vi "Autonomous Independent.vi"() -> ()   [LabVIEW 2017]
doc: "This VI is called when autonomous begins, and will automatically be terminated when autonomous ends. You can carry out timed or sensor driven robot movement independently without needing to return to the caller."
uses:
  <vilib>/Rock Robotics/WPI/Solenoid/WPI_SolenoidValue.ctl
  <vilib>/Rock Robotics/Network Tables/NT Read String.vi
  <vilib>/Rock Robotics/Network Tables/NT Read Numeric Array.vi
  <vilib>/Rock Robotics/Network Tables/NT Read String Array.vi
  <vilib>/Rock Robotics/WPI/Solenoid/WPI_SolenoidSetEnum.vi
  Robot Global Data.vi
panel:
  out "Setpoint2":dbl
  out "Setpoint":dbl
  in  "Z Drive PID Gains":T1
  # "Be sure to right-click and choose Data Operations>>Make Current Value default if you want to save the array values with the VI"
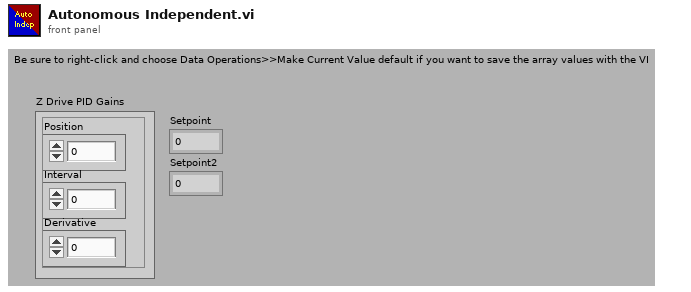
[diagram p1: front panel]
types:
  T1 = cluster{"Position":dbl, "Interval":dbl, "Derivative":dbl}
  T2 = typedef "WPI_SolenoidValue.ctl" = enum16{"Off", "On", "Forward", "Reverse"}
  T3 = enum16{"Front Left", "Front Right", "Back Left", "Back Right"}
  T4 = typedef "WPI_SolenoidDevRef.ctl" = cluster{"DevStatus":errorcluster, "Pneumatics Control Module":u8, "Forward Solenoid Channel":T5, "Reverse Solenoid Channel":T5}
  T5 = typedef "WPI_SolenoidChannel.ctl" = enum8{"Solenoid 0", "Solenoid 1", "Solenoid 2", "Solenoid 3", "Solenoid 4", "Solenoid 5", "Solenoid 6", "Solenoid 7", "Invalid"}
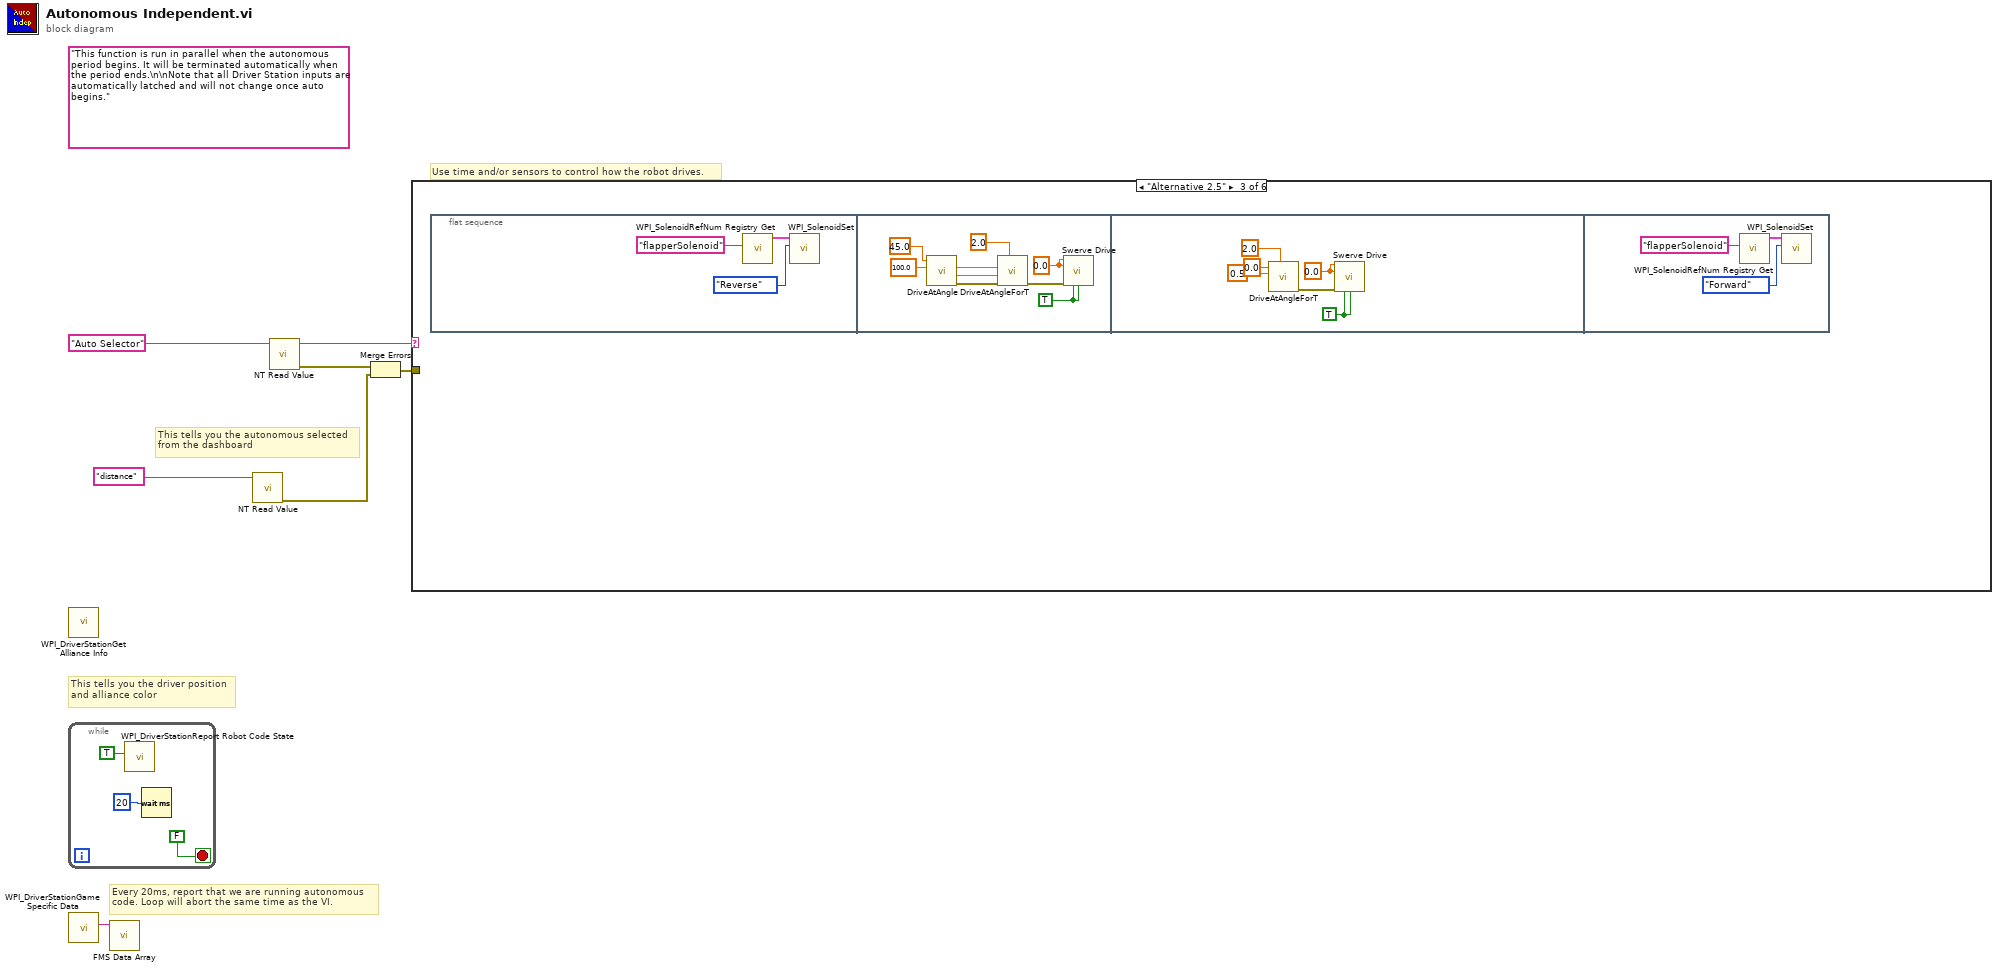
[diagram p0: block diagram]
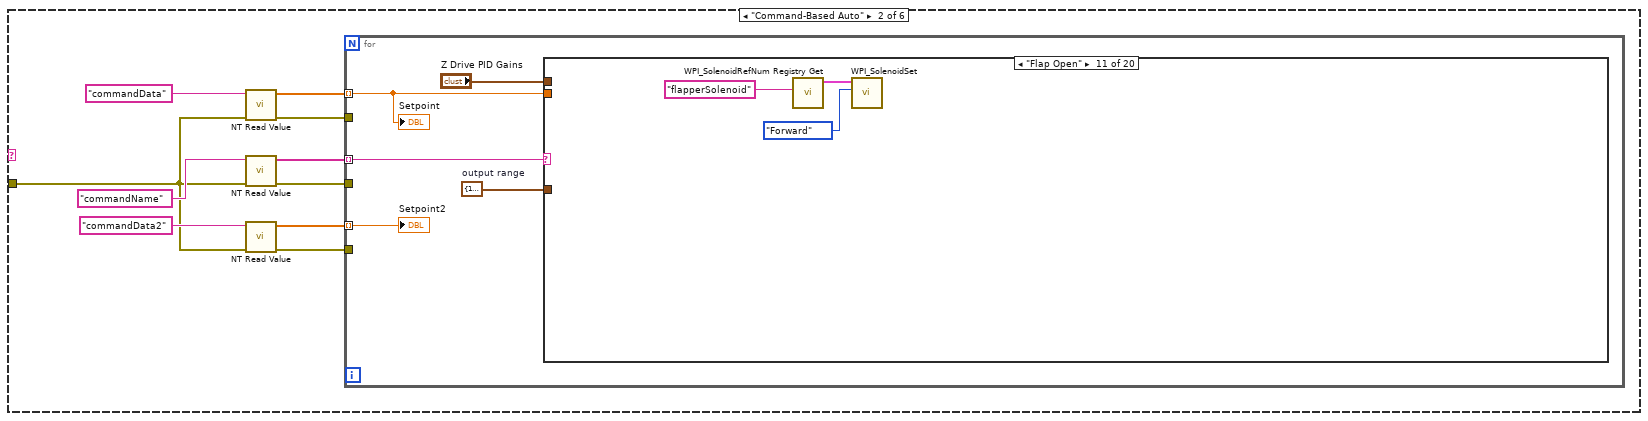
[diagram p3: hidden frame]
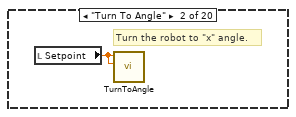
[diagram p5: hidden frame]
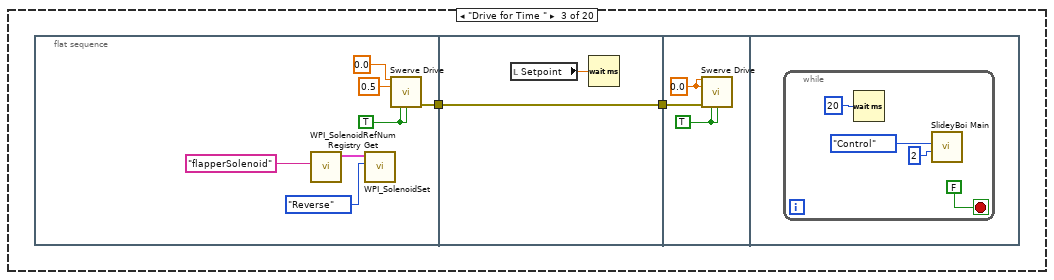
[diagram p6: hidden frame]
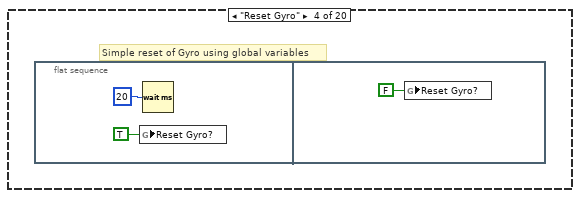
[diagram p7: hidden frame]
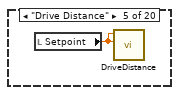
[diagram p8: hidden frame]
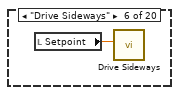
[diagram p9: hidden frame]
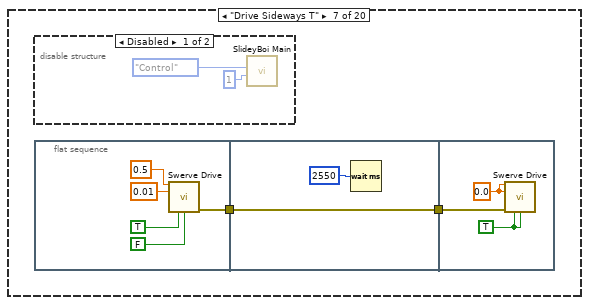
[diagram p10: hidden frame]
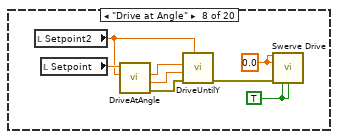
[diagram p12: hidden frame]
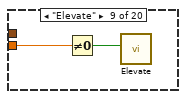
[diagram p13: hidden frame]
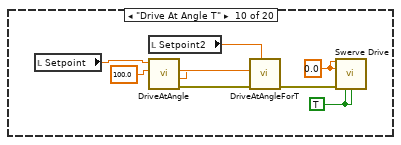
[diagram p14: hidden frame]
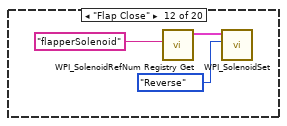
[diagram p15: hidden frame]
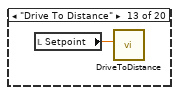
[diagram p16: hidden frame]
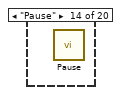
[diagram p17: hidden frame]
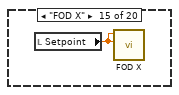
[diagram p18: hidden frame]
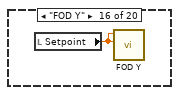
[diagram p19: hidden frame]
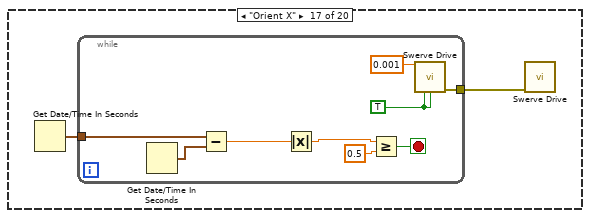
[diagram p20: hidden frame]
diagram:
  (unwired) "This function is run in parallel when the autonomous period begins. It will be terminated automatically when the period ends.\n\nNote that all Driver Station inputs are automatically latched and will not change once auto begins."
  # "This tells you the autonomous selected\nfrom the dashboard"
  # "Every 20ms, report that we are running autonomous\ncode. Loop will abort the same time as the VI."
  # "Use time and/or sensors to control how the robot drives."
  # "This tells you the driver position\nand alliance color"
  n1 = call <vilib>:"WPI_DriverStationGet Alliance Info.vi"() -> ()  [unwired: 12 out]
  n2 = while {
    stop <- FALSE stop-if-true
    n3 = call <vilib>:"WPI_DriverStationReport Robot Code State.vi"("Autonomous"=TRUE) -> ()  [unwired: 10 in, 1 out]
    n4 = Wait (ms)(milliseconds to wait=u32 20) -> ()  [unwired: 1 out]
  }
  n5 = call <vilib>:"WPI_DriverStationGame Specific Data.vi"() -> ("Game Specific Data"=w5:string)  [unwired: 11 in]
  n6 = call "FMS Data Array.vi"("Game Data"=w5) -> ()  [unwired: 8 in, 3 out]
  n7 = call-poly <vilib>:"NT Read Value.vi"("Name"="distance") -> ("error out"=w3:errorcluster)  [unwired: 9 in, 1 out]
  n8 = call-poly <vilib>:"NT Read Value.vi"("Name"="Auto Selector") -> ("error out"=w4:errorcluster, "String"=w6:string)  [unwired: 9 in]
  n9 = Merge Errors(w4, w3) -> (w1:errorcluster)
  n10 = case shown="\"Alternative 2.5\"" w6 {
    tunnel: w1 -> [_ w11 _ _ _ _]
    frame Default {
      # "You can put your main auto here, or you can right-click on the case and make any\nother frame be the default case."
      # "This is the frame that will execute if no selection is made, or if it is not recognized"
    }
    frame "Command-Based Auto" {
      n11 = call-poly <vilib>:"NT Read Value.vi"("error in"=w11, "Name"="commandData") -> ("error out"=w18:errorcluster, "Numeric Array"=w15:dbl[])  [unwired: 8 in]
      n12 = call-poly <vilib>:"NT Read Value.vi"("error in"=w11, "Name"="commandName") -> ("error out"=w17:errorcluster, "String Array"=w16:string[])  [unwired: 8 in]
      n13 = call-poly <vilib>:"NT Read Value.vi"("error in"=w11, "Name"="commandData2") -> ("error out"=w14:errorcluster, "Numeric Array"=w13:dbl[])  [unwired: 8 in]
      n14 = for {
        tunnel: w18 -> [_]
        tunnel: w17 -> [_]
        tunnel: w16 -> [w25] mode=indexing
        tunnel: w15 -> [w21] mode=indexing
        tunnel: w14 -> [_]
        tunnel: w13 -> [w24] mode=indexing
        w22 = cluster{dbl, dbl} {1.0, -1.0}  # output range
        n15 = case shown="\"Flap Open\"" w25 {
          tunnel: "Z Drive PID Gains" -> [_ _ _ _ _ _ _ _ _ _ _ _ _ _ _ _ _ _ _ _]
          tunnel: w22 -> [_ _ _ _ _ _ _ _ _ _ _ _ _ _ _ _ _ _ _ _]
          tunnel: w21 -> [_ _ _ _ _ _ _ _ w73 _ _ _ _ _ _ _ _ _ _ _]
          frame Default {
          }
          frame "Turn To Angle" {
            # "Turn the robot to \"x\" angle."
            n16 = local read "Setpoint"() -> (w26:dbl)
            n17 = call "TurnToAngle.vi"(10:"Target Angle"=w26, 11:"Target Angle"=w26) -> ()  [unwired: 9 in, 1 out]
          }
          frame "Drive for Time " {
            n18 = flat-sequence {
              tunnel: [w32] -> w28
              tunnel: [w37] -> w27
              tunnel: w28 -> [w37]
              tunnel: w27 -> [w39]
              frame #0 {
                w33 = TRUE ("Autonomous?")
                n19 = call <vilib>:"WPI_SolenoidRefNum Registry Get.vi"("refnum name"="flapperSolenoid") -> ("SolenoidDevRef"=w31:T4)  [unwired: 9 in, 1 out]
                n20 = call-poly <vilib>:"WPI_SolenoidSet.vi"("Value"=WPI_SolenoidValue."Reverse", "SolenoidDevRef"=w31) -> ()  [unwired: 8 in, 2 out]
                n21 = call "Swerve Drive.vi"("X"=0.0, "Y"=0.5, "Robot Centric?"=w33, "Autonomous?"=w33) -> ("Error Out"=w32:errorcluster)  [unwired: 7 in, 4 out]
              }
              frame #1 {
                n22 = local read "Setpoint"() -> (w36:dbl)
                n23 = Wait (ms)(milliseconds to wait=w36) -> ()  [unwired: 1 out]
              }
              frame #2 {
                w38 = TRUE ("Robot Centric?")
                w40 = 0.0 ("X")
                n24 = call "Swerve Drive.vi"("X"=w40, "Y"=w40, "Error In"=w39, "Robot Centric?"=w38, "Autonomous?"=w38) -> ()  [unwired: 6 in, 5 out]
              }
              frame #3 {
                n25 = while {
                  stop <- FALSE stop-if-true
                  n26 = Wait (ms)(milliseconds to wait=u32 20) -> ()  [unwired: 1 out]
                  n27 = call "SlideyBoi Main.vi"("Control Option"=u32 2, "Control Mode"=enum16{"Open", "Control"}."Control") -> ()  [unwired: 10 in]
                }
              }
            }
          }
          frame "Reset Gyro" {
            # "Simple reset of Gyro using global variables"
            n28 = flat-sequence {
              frame #0 {
                n29 = global write "Robot Global Data.vi" "Reset Gyro?"(TRUE ("Enable Vision")) -> ()
                n30 = Wait (ms)(milliseconds to wait=u32 20) -> ()  [unwired: 1 out]
              }
              frame #1 {
                n31 = global write "Robot Global Data.vi" "Reset Gyro?"(FALSE ("Reset Gyro?")) -> ()
              }
            }
          }
          frame "Drive Distance" {
            n32 = local read "Setpoint"() -> (w48:dbl)
            n33 = call "DriveDistance.vi"(10:"Setpoint"=w48, 11:"Setpoint"=w48) -> ()  [unwired: 10 in]
          }
          frame "Drive Sideways" {
            n34 = local read "Setpoint"() -> (w49:dbl)
            n35 = call "Drive Sideways.vi"("Setpoint"=w49) -> ()  [unwired: 10 in]
          }
          frame "Drive Sideways T" {
            n36 = disable-structure shown="Disabled" {
              frame Disabled {
                n37 = call "SlideyBoi Main.vi"("Control Option"=u32 1, "Control Mode"=enum16{"Open", "Control"}."Control") -> ()  [unwired: 10 in]
              }
              frame Enabled {
              }
            }
            n38 = flat-sequence {
              tunnel: [w55] -> w51
              tunnel: w51 -> [w59]
              tunnel: [w59] -> w50
              tunnel: w50 -> [w61]
              frame #0 {
                n39 = call "Swerve Drive.vi"("X"=0.5, "Y"=0.01, "Robot Centric?"=TRUE, "Autonomous?"=FALSE) -> ("Error Out"=w55:errorcluster)  [unwired: 7 in, 4 out]
              }
              frame #1 {
                n40 = Wait (ms)(milliseconds to wait=u32 2550) -> ()  [unwired: 1 out]
              }
              frame #2 {
                w62 = TRUE
                w63 = 0.0 ("X")
                n41 = call "Swerve Drive.vi"("X"=w63, "Y"=w63, "Error In"=w61, "Robot Centric?"=w62, "Autonomous?"=w62) -> ()  [unwired: 6 in, 5 out]
              }
            }
          }
          frame "Drive at Angle" {
            w65 = TRUE ("Robot Centric?")
            w70 = 0.0 ("X")
            n42 = local read "Setpoint2"() -> (w64:dbl)
            n43 = local read "Setpoint"() -> (w68:dbl)
            n44 = call "DriveAtAngle.vi"("Target Angle"=w68, "Distance"=w64) -> ("x"=w66:dbl, "y"=w67:dbl, "Error Out"=w71:errorcluster)  [unwired: 5 in, 1 out]
            n45 = call "DriveUntilY.vi"("Stop  Distance"=w64, "error in"=w71, "y"=w67, "x"=w66) -> ("error out"=w69:errorcluster)  [unwired: 7 in]
            n46 = call "Swerve Drive.vi"("X"=w70, "Y"=w70, "Error In"=w69, "Robot Centric?"=w65, "Autonomous?"=w65) -> ()  [unwired: 6 in, 5 out]
          }
          frame "Elevate" {
            n47 = Not Equal To 0?(x=w73) -> (x != 0?=w72:bool)
            n48 = call "Elevate.vi"("Reverse"=w72) -> ()  [unwired: 11 in]
          }
          frame "Drive At Angle T" {
            w78 = 0.0 ("X")
            w77 = TRUE ("Robot Centric?")
            n49 = local read "Setpoint"() -> (w82:dbl)
            n50 = local read "Setpoint2"() -> (w76:dbl)
            n51 = call "DriveAtAngle.vi"("Target Angle"=w82, "Distance"=100.0) -> ("x"=w81:dbl, "y"=w80:dbl, "Error Out"=w75:errorcluster)  [unwired: 5 in, 1 out]
            n52 = call "DriveAtAngleForT.vi"("time(sec)"=w76, "Error In"=w75, "y"=w80, "x"=w81) -> ("Error Out"=w79:errorcluster)  [unwired: 7 in]
            n53 = call "Swerve Drive.vi"("X"=w78, "Y"=w78, "Error In"=w79, "Robot Centric?"=w77, "Autonomous?"=w77) -> ()  [unwired: 6 in, 5 out]
          }
          frame "Flap Open" {
            n54 = call <vilib>:"WPI_SolenoidRefNum Registry Get.vi"("refnum name"="flapperSolenoid") -> ("SolenoidDevRef"=w84:T4)  [unwired: 9 in, 1 out]
            n55 = call-poly <vilib>:"WPI_SolenoidSet.vi"("Value"=WPI_SolenoidValue."Forward", "SolenoidDevRef"=w84) -> ()  [unwired: 8 in, 2 out]
          }
          frame "Flap Close" {
            n56 = call <vilib>:"WPI_SolenoidRefNum Registry Get.vi"("refnum name"="flapperSolenoid") -> ("SolenoidDevRef"=w88:T4)  [unwired: 9 in, 1 out]
            n57 = call-poly <vilib>:"WPI_SolenoidSet.vi"("Value"=WPI_SolenoidValue."Reverse", "SolenoidDevRef"=w88) -> ()  [unwired: 8 in, 2 out]
          }
          frame "Drive To Distance" {
            n58 = local read "Setpoint"() -> (w89:dbl)
            n59 = call "DriveToDistance.vi"("Setpoint"=w89) -> ()  [unwired: 10 in, 1 out]
          }
          frame "Pause" {
            n60 = call "Pause.vi"() -> ()  [unwired: 11 in, 1 out]
          }
          frame "FOD X" {
            n61 = local read "Setpoint"() -> (w90:dbl)
            n62 = call "FOD X.vi"(10:"Setpoint"=w90, 11:"Setpoint"=w90) -> ()  [unwired: 10 in]
          }
          frame "FOD Y" {
            n63 = local read "Setpoint"() -> (w91:dbl)
            n64 = call "FOD Y.vi"(10:"Setpoint"=w91, 11:"Setpoint"=w91) -> ()  [unwired: 10 in]
          }
          frame "Orient X" {
            n65 = Get Date/Time In Seconds() -> (seconds since 1Jan1904=w93:timestamp)
            n66 = while {
              tunnel: w93 -> [w101]
              tunnel: [w96] -> w92
              stop <- w97 stop-if-true
              w94 = TRUE ("Robot Centric?")
              n67 = Get Date/Time In Seconds() -> (seconds since 1Jan1904=w102:timestamp)
              n68 = Subtract(x=w101, y=w102) -> (x-y=w100:dbl)
              n69 = Absolute Value(x=w100) -> (abs(x)=w99:dbl)
              n70 = Greater Or Equal?(x=w99, y=0.5) -> (x >= y?=w97:bool)
              n71 = call "Swerve Drive.vi"("X"=0.001, "Robot Centric?"=w94, "Autonomous?"=w94) -> ("Error Out"=w96:errorcluster)  [unwired: 8 in, 4 out]
            }
            n72 = call "Swerve Drive.vi"("Error In"=w92) -> ()  [unwired: 10 in, 5 out]
          }
          frame "Orient Y" {
            n73 = Get Date/Time In Seconds() -> (seconds since 1Jan1904=w104:timestamp)
            n74 = while {
              tunnel: w104 -> [w112]
              tunnel: [w107] -> w103
              stop <- w108 stop-if-true
              w105 = TRUE ("Robot Centric?")
              n75 = Get Date/Time In Seconds() -> (seconds since 1Jan1904=w113:timestamp)
              n76 = Subtract(x=w112, y=w113) -> (x-y=w111:dbl)
              n77 = Absolute Value(x=w111) -> (abs(x)=w110:dbl)
              n78 = Greater Or Equal?(x=w110, y=0.5) -> (x >= y?=w108:bool)
              n79 = call "Swerve Drive.vi"("X"=0.001, "Robot Centric?"=w105, "Autonomous?"=w105) -> ("Error Out"=w107:errorcluster)  [unwired: 8 in, 4 out]
            }
            n80 = call "Swerve Drive.vi"("Error In"=w103) -> ()  [unwired: 10 in, 5 out]
          }
          frame "Collide Drive X" {
            n81 = local read "Setpoint"() -> (w114:dbl)
            n82 = call "CollideDriveX.vi"(10:"Setpoint"=w114, 11:"Setpoint"=w114) -> ()  [unwired: 10 in]
          }
          frame "Collide Drive Y" {
            n83 = local read "Setpoint"() -> (w115:dbl)
            n84 = call "CollideDriveY.vi"(10:"Setpoint"=w115, 11:"Setpoint"=w115) -> ()  [unwired: 10 in]
          }
        }
        "Setpoint" <- w21
        "Setpoint2" <- w24
      }
    }
    frame "Alternative 2.5" {
      n85 = flat-sequence {
        frame #0 {
          n86 = call <vilib>:"WPI_SolenoidRefNum Registry Get.vi"("refnum name"="flapperSolenoid") -> ("SolenoidDevRef"=w116:T4)  [unwired: 9 in, 1 out]
          n87 = call-poly <vilib>:"WPI_SolenoidSet.vi"("Value"=WPI_SolenoidValue."Reverse", "SolenoidDevRef"=w116) -> ()  [unwired: 8 in, 2 out]
        }
        frame #1 {
          w124 = 0.0 ("X")
          w123 = TRUE ("Robot Centric?")
          n88 = call "DriveAtAngle.vi"("Target Angle"=45.0, "Distance"=100.0) -> ("x"=w127:dbl, "y"=w126:dbl, "Error Out"=w122:errorcluster)  [unwired: 5 in, 1 out]
          n89 = call "DriveAtAngleForT.vi"("time(sec)"=2.0, "Error In"=w122, "y"=w126, "x"=w127) -> ("Error Out"=w125:errorcluster)  [unwired: 7 in]
          n90 = call "Swerve Drive.vi"("X"=w124, "Y"=w124, "Error In"=w125, "Robot Centric?"=w123, "Autonomous?"=w123) -> ()  [unwired: 6 in, 5 out]
        }
        frame #2 {
          w132 = 0.0 ("X")
          w130 = TRUE ("Robot Centric?")
          n91 = call "DriveAtAngleForT.vi"("time(sec)"=2.0, "y"=0.5, "x"=0.0) -> ("Error Out"=w131:errorcluster)  [unwired: 8 in]
          n92 = call "Swerve Drive.vi"("X"=w132, "Y"=w132, "Error In"=w131, "Robot Centric?"=w130, "Autonomous?"=w130) -> ()  [unwired: 6 in, 5 out]
        }
        frame #3 {
          n93 = call <vilib>:"WPI_SolenoidRefNum Registry Get.vi"("refnum name"="flapperSolenoid") -> ("SolenoidDevRef"=w135:T4)  [unwired: 9 in, 1 out]
          n94 = call-poly <vilib>:"WPI_SolenoidSet.vi"("Value"=WPI_SolenoidValue."Forward", "SolenoidDevRef"=w135) -> ()  [unwired: 8 in, 2 out]
        }
      }
    }
    frame "Swerve Calibration" {
      n95 = call "Swerve Calibrate.vi"("Wheel Corner"=T3."Front Left") -> ("error out"=w142:errorcluster)  [unwired: 10 in]
      n96 = call "Swerve Calibrate.vi"("error in (no error)"=w142, "Wheel Corner"=T3."Front Right") -> ("error out"=w140:errorcluster)  [unwired: 9 in]
      n97 = call "Swerve Calibrate.vi"("error in (no error)"=w140, "Wheel Corner"=T3."Back Left") -> ("error out"=w138:errorcluster)  [unwired: 9 in]
      n98 = call "Swerve Calibrate.vi"("error in (no error)"=w138, "Wheel Corner"=T3."Back Right") -> ()  [unwired: 9 in, 1 out]
    }
    frame "Alternative 1" {
      n99 = flat-sequence {
        tunnel: [w149] -> w144
        tunnel: [w154] -> w145
        tunnel: w144 -> [w154]
        tunnel: w145 -> [w156]
        frame #0 {
          w150 = TRUE ("Autonomous?")
          n100 = call "Swerve Drive.vi"("X"=0.0, "Y"=0.5, "Robot Centric?"=w150, "Autonomous?"=w150) -> ("Error Out"=w149:errorcluster)  [unwired: 7 in, 4 out]
          n101 = call <vilib>:"WPI_SolenoidRefNum Registry Get.vi"("refnum name"="flapperSolenoid") -> ("SolenoidDevRef"=w148:T4)  [unwired: 9 in, 1 out]
          n102 = call-poly <vilib>:"WPI_SolenoidSet.vi"("Value"=WPI_SolenoidValue."Reverse", "SolenoidDevRef"=w148) -> ()  [unwired: 8 in, 2 out]
        }
        frame #1 {
          n103 = Wait (ms)(milliseconds to wait=u32 2400) -> ()  [unwired: 1 out]
        }
        frame #2 {
          w155 = TRUE ("Robot Centric?")
          w157 = 0.0 ("X")
          n104 = call "Swerve Drive.vi"("X"=w157, "Y"=w157, "Error In"=w156, "Robot Centric?"=w155, "Autonomous?"=w155) -> ()  [unwired: 6 in, 5 out]
        }
      }
    }
    frame "Unwind Motors" {
      n105 = call "Motor Unwind.vi"("Encoder Refnum"="backRightEnc" ("refnum name"), "Switch Refnum"="backRightSwitch", "Motor Refnum"="backRightRotation" ("refnum name")) -> ()  [unwired: 9 in]
      n106 = call "Motor Unwind.vi"("Encoder Refnum"="frontRightEnc" ("refnum name"), "Switch Refnum"="frontRightSwitch", "Motor Refnum"="frontRightRotation" ("refnum name")) -> ()  [unwired: 9 in]
      n107 = call "Motor Unwind.vi"("Encoder Refnum"="frontLeftEnc" ("refnum name"), "Switch Refnum"="frontLeftSwitch", "Motor Refnum"="frontLeftRotation" ("refnum name")) -> ()  [unwired: 9 in]
      n108 = call "Motor Unwind.vi"("Encoder Refnum"="backLeftEnc" ("refnum name"), "Switch Refnum"="backLeftSwitch", "Motor Refnum"="backLeftRotation" ("refnum name")) -> ()  [unwired: 9 in]
    }
  }
